vi "Register Channel.vi"(8 "error in (no error)":errorcluster, 10 "Channel":refnum<class "CIFChannels.lvclass">, 11 "CIFCorePlugin in":refnum<class "CIFCorePlugin.lvclass">) -> (0 "error out":errorcluster, 3 "CIFCorePlugin out":refnum<class "CIFCorePlugin.lvclass">)   [LabVIEW 2021, in "CIFCorePlugin.lvclass"]
uses:
  CIFCorePlugin.lvclass
  Channels/CIFChannels/CIFChannels.lvclass
  CIFCorePlugin.lvclass/CIFCorePlugin.ctl
  Channels/CIFChannels/CIFChannels.lvclass/CIFChannels.ctl
  Channels/CIFChannelMng/CIFChannelMng.lvclass/CIFChannelMng.ctl
  CIFUtilities/CIFClocks/SubVIs/Add Error.vi
  Channels/CIFChannels/Accessors/Read Name.vi
  Channels/CIFChannels/Accessors/Read Custom Config Data.vi
  Channels/CIFChannels/Accessors/Read Channel Class.vi
  Channels/CIFChannels/Accessors/Read Direction.vi
  Common/Utilities/Append Error Location.vi
  Channels/CIFChannelMng/CIFChannelMng.lvclass
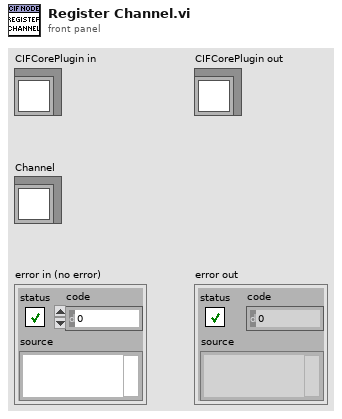
[diagram p1: front panel]
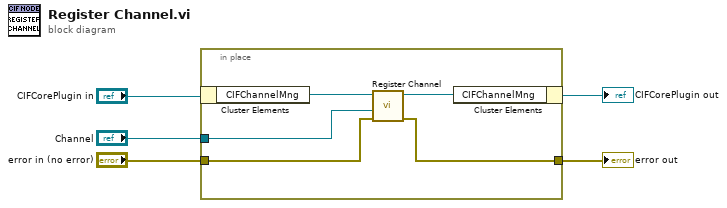
[diagram p0: block diagram]
diagram:
  n1 = in-place {
    in-place-border: "error in (no error)" -> [w8]
    in-place-border: [w7] -> w1
    in-place-border: "Channel" -> [w6]
    n2 = in-place-cluster #1("CIFCorePlugin in") -> ("CIFChannelMng"=w10:refnum<class "CIFChannelMng.lvclass">)
    n3 = call "Register Channel.vi"("error in (no error)"=w8, "Channel"=w6, "CIFChannelMng in"=w10) -> ("error out"=w7:errorcluster, "CIFChannelMng out"=w9:refnum<class "CIFChannelMng.lvclass">)  [unwired: 7 in]
    n4 = in-place-cluster #1("CIFChannelMng"=w9) -> (→"CIFCorePlugin out":refnum<class "CIFCorePlugin.lvclass">)
  }
  "error out" <- w1
